vi "ReadUART.vi"(8 "error in (no error)":errorcluster, 11 "GiaoTiep in":refnum<class "GiaoTiepUART.lvclass">) -> (0 "error out":errorcluster, 1 "milisecondGetData":dbl, 2 "read buffer":string, 3 "GiaoTiep out":refnum<class "GiaoTiepUART.lvclass">)   [LabVIEW 2014, in "LibraryGcode.lvlib" / "GiaoTiepUART.lvclass"]
uses:
  GiaoTiepUART.lvclass
  GiaoTiepUART.lvclass/GiaoTiepUART.ctl
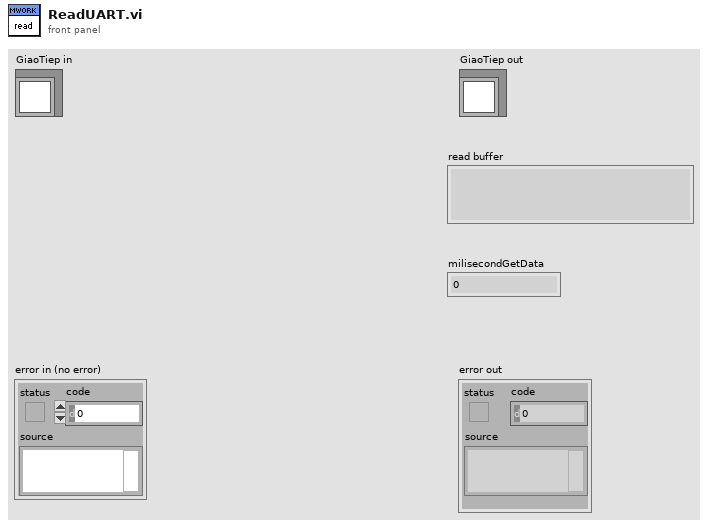
[diagram p1: front panel]
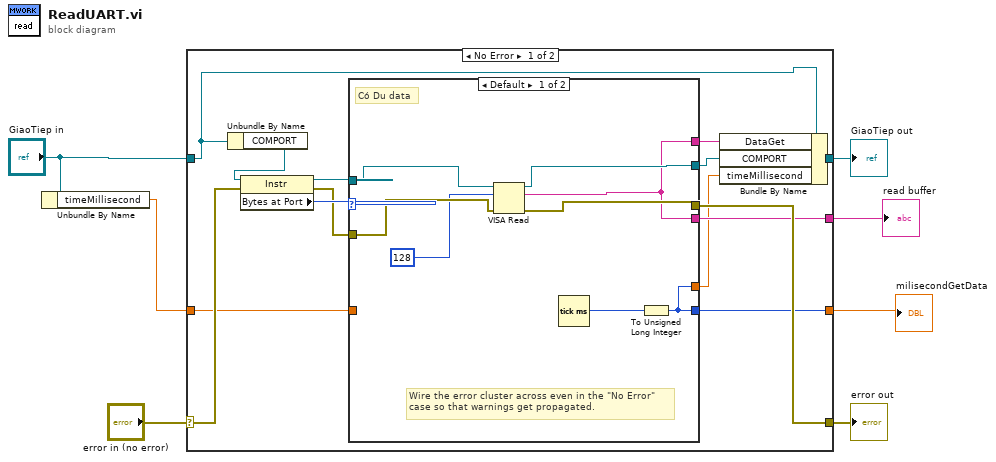
[diagram p0: block diagram]
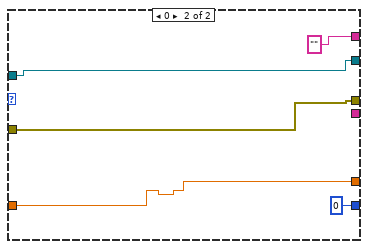
[diagram p2: hidden frame]
diagram:
  n1 = Unbundle By Name("GiaoTiep in") -> ("timeMillisecond"=w1:dbl)
  n2 = case shown="No Error" "error in (no error)" {
    selector: "error in (no error)" -> [w18 w37]
    tunnel: [w19 w37] -> w6
    tunnel: [w15 w36] -> w5
    tunnel: "GiaoTiep in" -> [w9 w36]
    tunnel: [w14 _] -> w4
    tunnel: [w12 w35] -> w3
    tunnel: w1 -> [w13 w35]
    frame No Error {
      # "Wire the error cluster across even in the \"No Error\"\ncase so that warnings get propagated."
      n3 = Unbundle By Name(w9) -> ("COMPORT"=w17:refnum<visa-resource-name>)
      n4 = property class="Instr"(reference=w17, error in=w18) -> (reference out=w21:refnum<visa-resource-name>, error out=w10:errorcluster, "Bytes at Port"=w20:u32)
      n5 = case shown="Default" w20 {
        tunnel: w21 -> [w27 w34]
        tunnel: w10 -> [w26 w33]
        tunnel: [w28 w33] -> w19
        tunnel: [w29 w34] -> w16
        tunnel: [w24 _] -> w14
        tunnel: [w22 u32 0 ("millisecond timer value")] -> w12
        tunnel: w13 -> [_ w30]
        tunnel: [w22 w30] -> w11
        tunnel: [w24 "" ("DataGet")] -> w8
        frame Default {
          # "Có Du data"
          n6 = VISA Read(VISA resource name=w27, byte count=u32 128, error in (no error)=w26) -> (VISA resource name out=w29:refnum<visa-resource-name>, read buffer=w24:string, error out=w28:errorcluster)  [unwired: 1 out]
          n7 = Tick Count (ms)() -> (millisecond timer value=w23:u32)
          n8 = To Unsigned Long Integer(number=w23) -> (unsigned 32bit integer=w22:u32)
        }
        frame 0 {
        }
      }
      n9 = Bundle By Name(cluster=w9, "DataGet"=w8, "COMPORT"=w16, "timeMillisecond"=w11) -> (w15:refnum<class "GiaoTiepUART.lvclass">)
    }
    frame Error {
    }
  }
  "error out" <- w6
  "GiaoTiep out" <- w5
  "read buffer" <- w4
  "milisecondGetData" <- w3
